vi "closed_loop.vi"() -> ()   [LabVIEW 2018]
uses:
  Controls/StatisticsData.ctl
  Classes/WavefrontCorrector/WavefrontCorrector.lvclass
  Classes/SlopesPostProcessorList/SlopesPostProcessorList.lvclass
  Classes/CorrectionDataManager/CorrectionDataManager.lvclass
  Classes/Camera/Camera.lvclass
  Classes/HasoEngine/HasoEngine.lvclass
  Classes/WavefrontCorrectorSet/WavefrontCorrectorSet.lvclass
  Classes/HasoData/HasoData.lvclass
  Classes/HasoSlopes/HasoSlopes.lvclass
  Classes/Image/Image.lvclass
  Classes/Phase/Phase.lvclass
  Classes/Pupil/Pupil.lvclass
  Classes/ComputePhaseSet/ComputePhaseSet.lvclass
  Classes/ClosedLoopSmoothing/ClosedLoopSmoothing.lvclass
  Controls/WavefrontReconstructionMode.ctl
  Controls/SlopesPostProcessorList - Filter.ctl
  Controls/InteractionMatrixToCommandMatrixParameters.ctl
panel:
  in  "init_state_from_config_file":bool
  out "Gain out":dbl min=0.0 max=1.0
  in  "Gain in":dbl min=0.0 max=1.0
  in  "Init":bool
  in  "Start Loop":bool
  in  "Exit":bool
  in  "Stop Loop":bool
  in  "error in (no error)":errorcluster
  out "Phase values":sgl[][](graph)
  out "Phase statistics":T1
  out "Camera image":u32[][](graph)
  in  "Interaction matrix file path":path
  out "error out":errorcluster
  out "ActuatorsNumber":i32
  in  "Wavefront configuration file path":path
  in  "Haso configuration file path":path
  # "This example is Hardware-dependant, \nplease use your own Haso and corrector configuration file and acquisition system, as well as your correction data backup file.\nIf you don't have a correction data backup file, please run the correction data example."
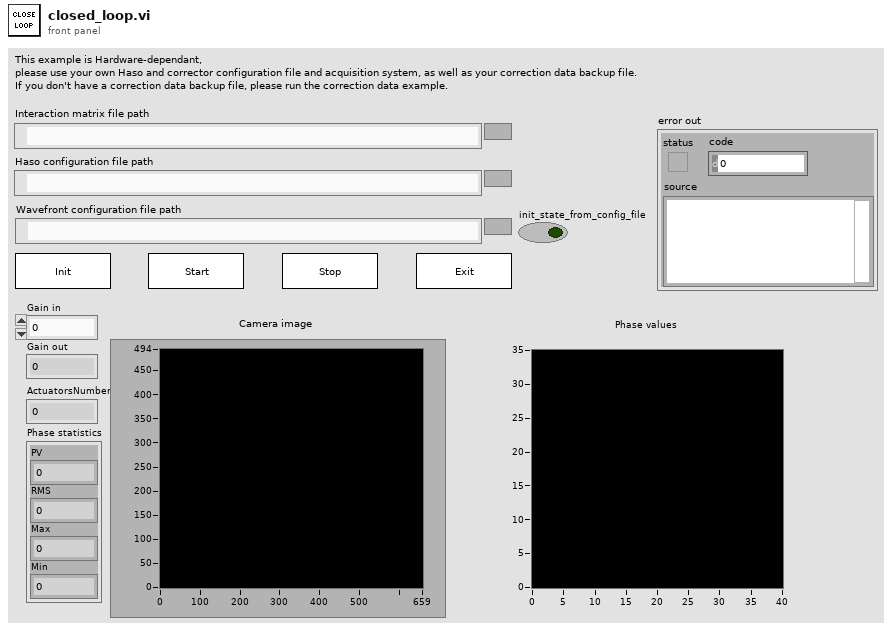
[diagram p1: front panel]
types:
  T1 = typedef "StatisticsData.ctl" = cluster{"PV":sgl, "RMS":dbl, "Max":sgl, "Min":sgl}
  T2 = typedef "WavefrontReconstructionMode.ctl" = enum16{"None", "Modal_Legendre", "Modal_Zernike", "Zonal", "Modal_Zonal_Zernike", "Modal_Zonal_Legendre"}
  T3 = typedef "SlopesPostProcessorList - Filter.ctl" = cluster{"tiltx":bool, "tilty":bool, "curv":bool, "astig0":bool, "astig45":bool, "others":bool}
  T4 = typedef "InteractionMatrixToCommandMatrixParameters.ctl" = cluster{"Number of kept modes":i32, "Tilt filtering":bool}
  T5 = typedef "CasaoManagerGeneralSpecifications.ctl" = cluster{"Wavefront corrector name":string, "Wavefront corrector serial number":string, "Nb actuators":i32, "HASO serial number":string, "Dimension_um":T6}
  T6 = typedef "General dimensions definition.ctl" = cluster{"Size":T7, "Step":T8}
  T7 = typedef "Point2D.ctl" = cluster{"X":u32, "Y":u32}
  T8 = typedef "Point2Df.ctl" = cluster{"X":sgl, "Y":sgl}
  T9 = typedef "Data alignment enum.ctl" = enum16{"8", "16", "32"}
  T10 = typedef "Wavefront Corrector states - ONE.ctl" = cluster{"Max":sgl, "Min":sgl, "Validity":enum16{"valid", "fixed", "invalid"}, "Fixed_Position":sgl}
  T11 = typedef "Wavefront Corrector Position.ctl" = sgl[]
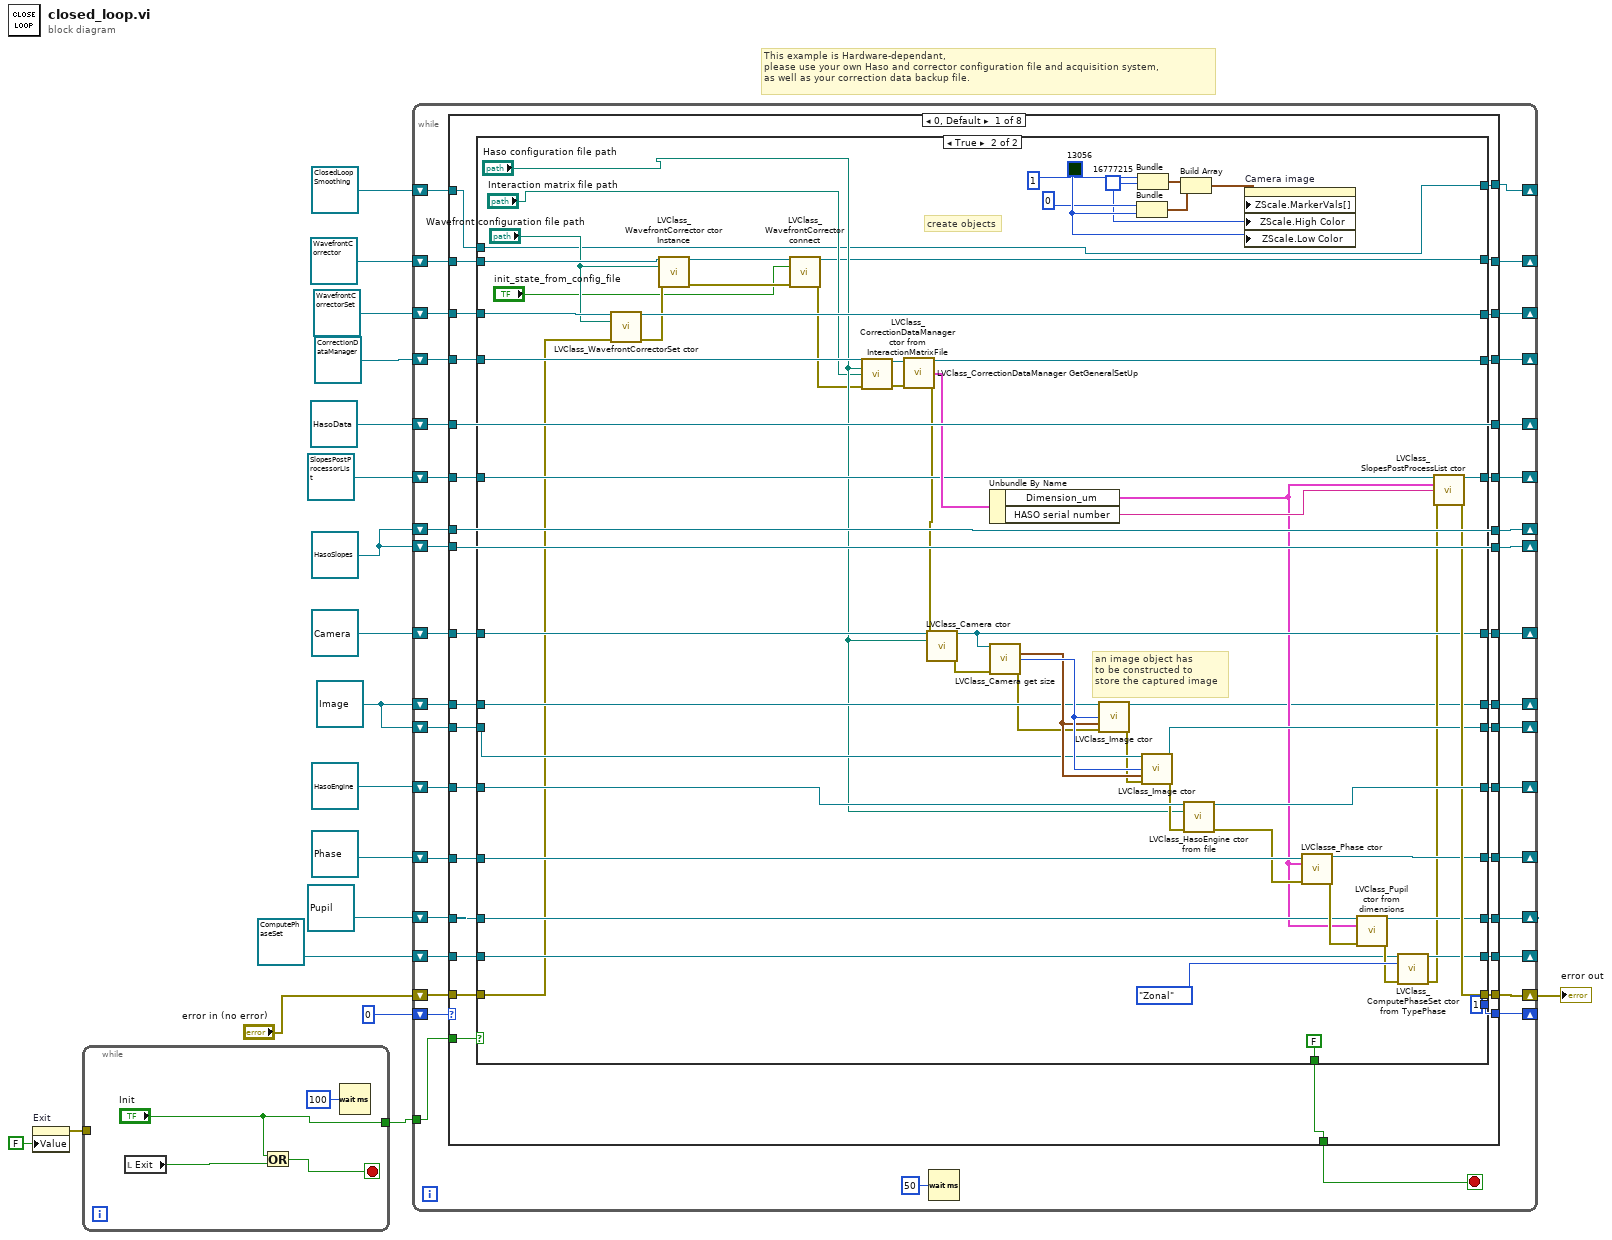
[diagram p0: block diagram]
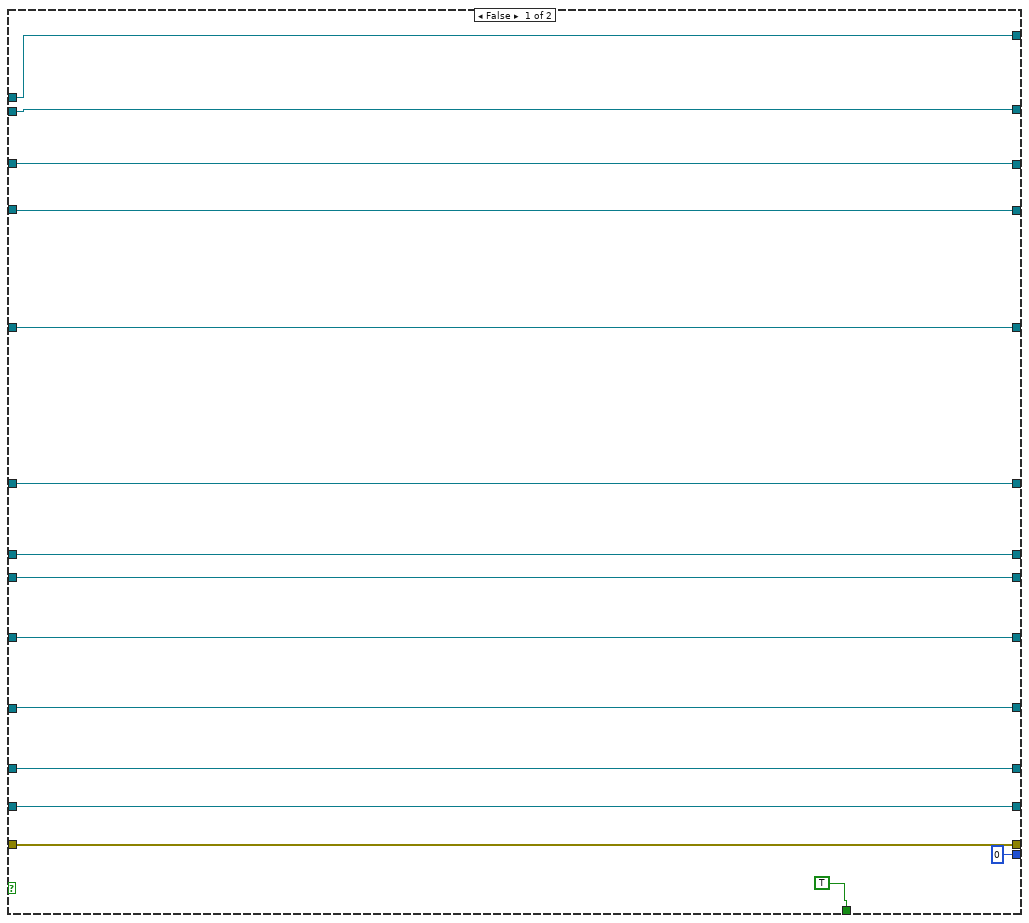
[diagram p2: hidden frame]
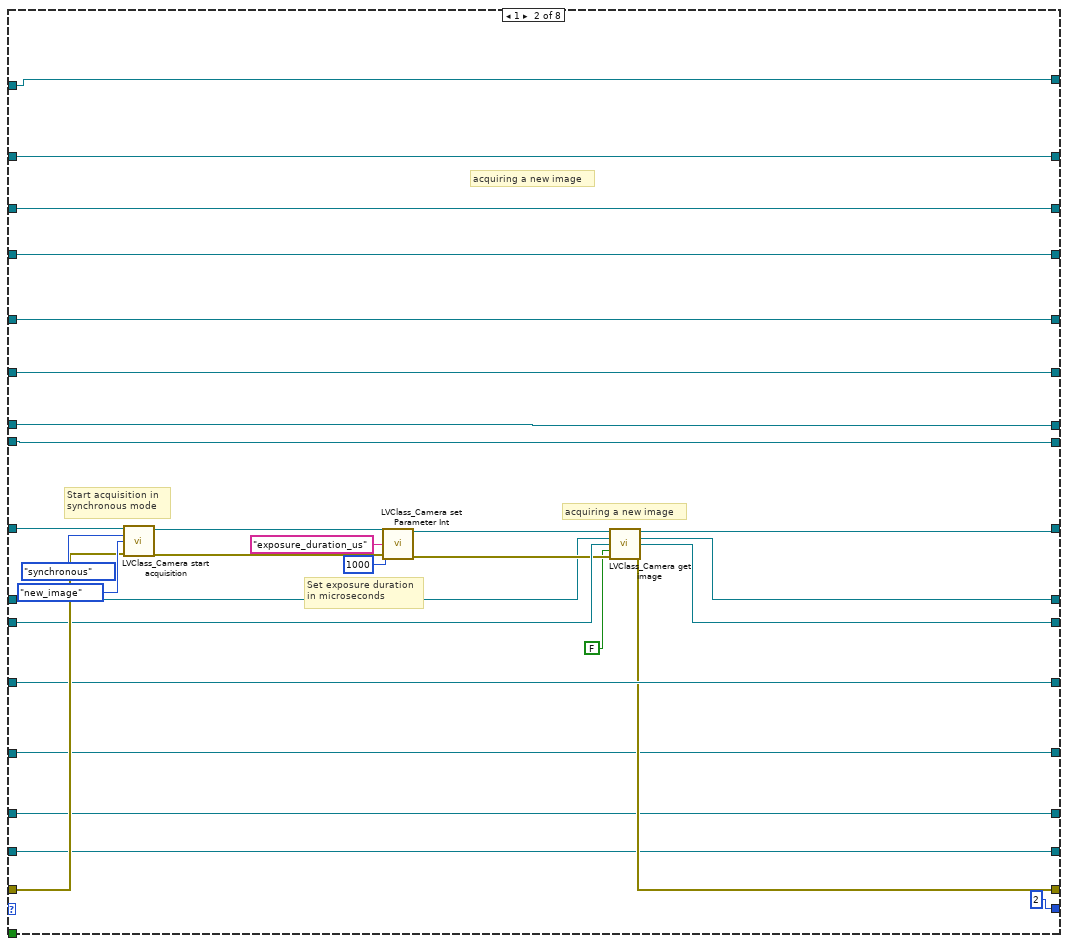
[diagram p3: hidden frame]
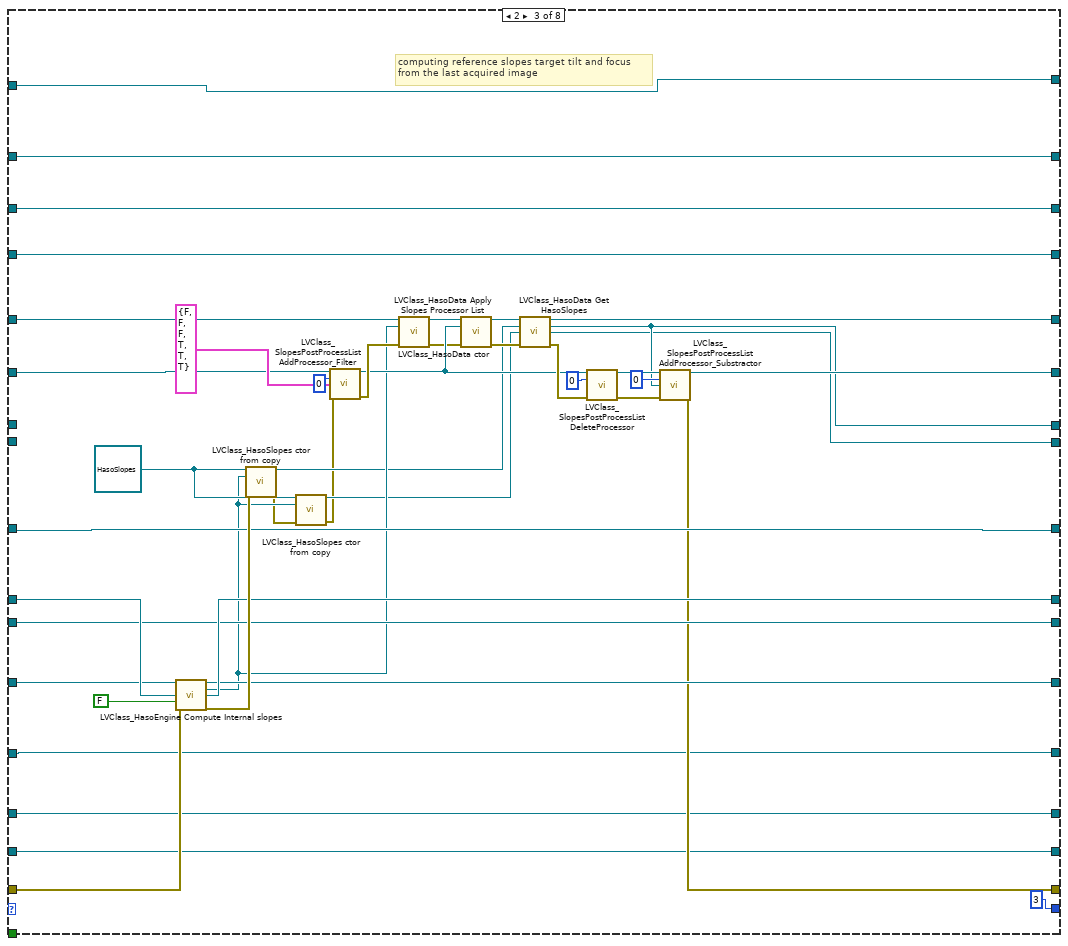
[diagram p4: hidden frame]
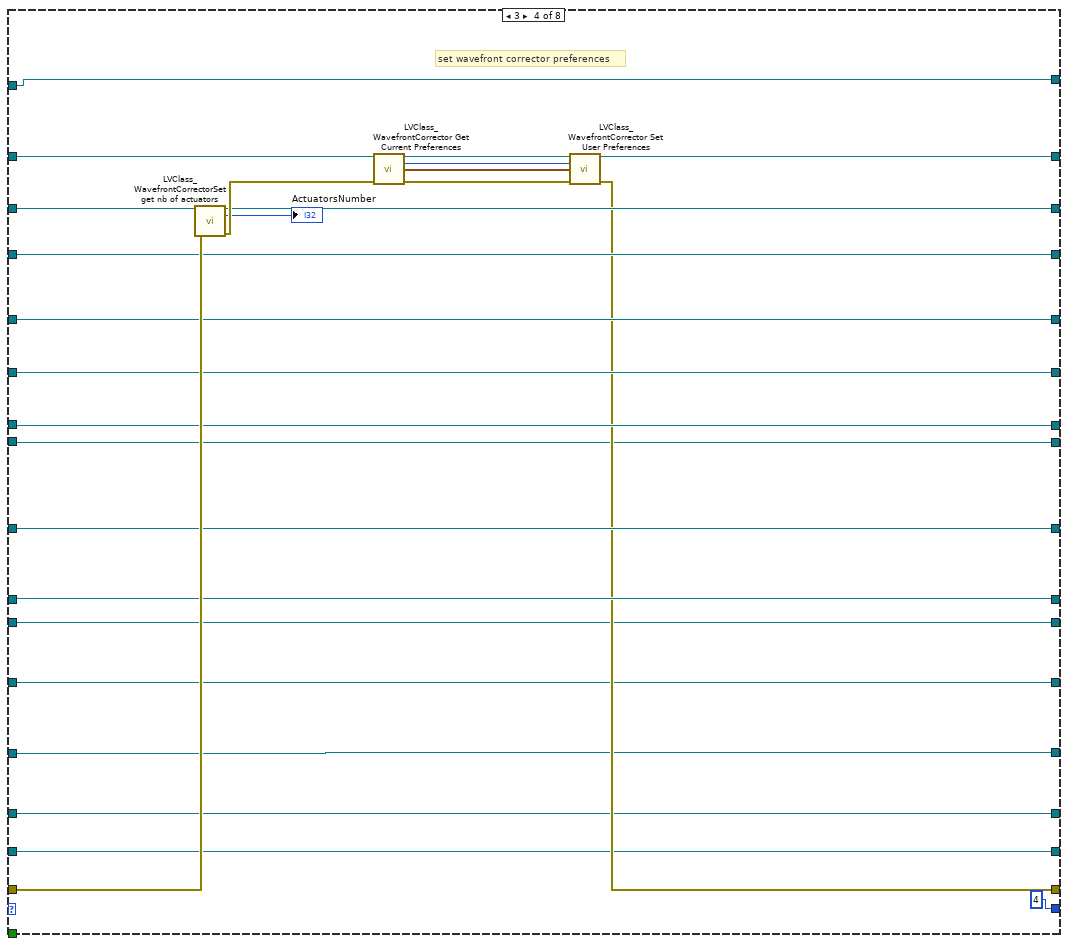
[diagram p5: hidden frame]
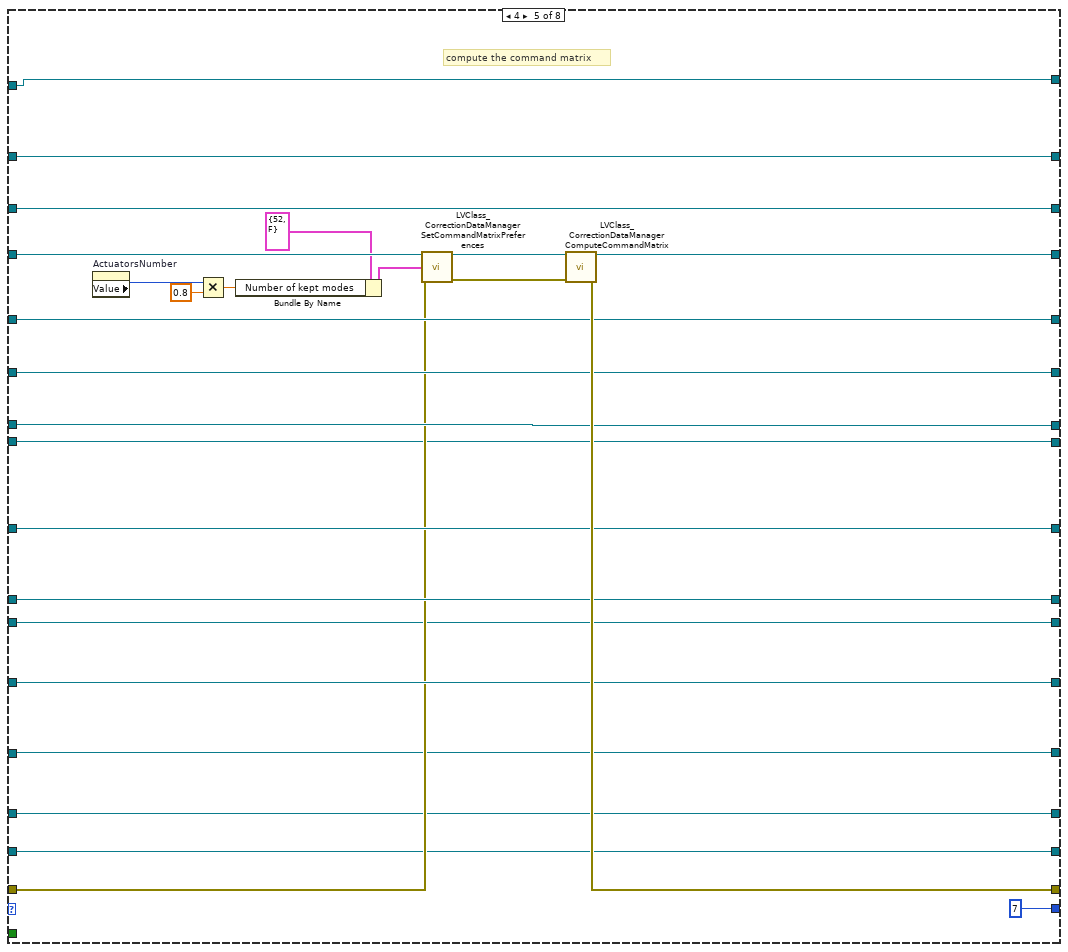
[diagram p6: hidden frame]
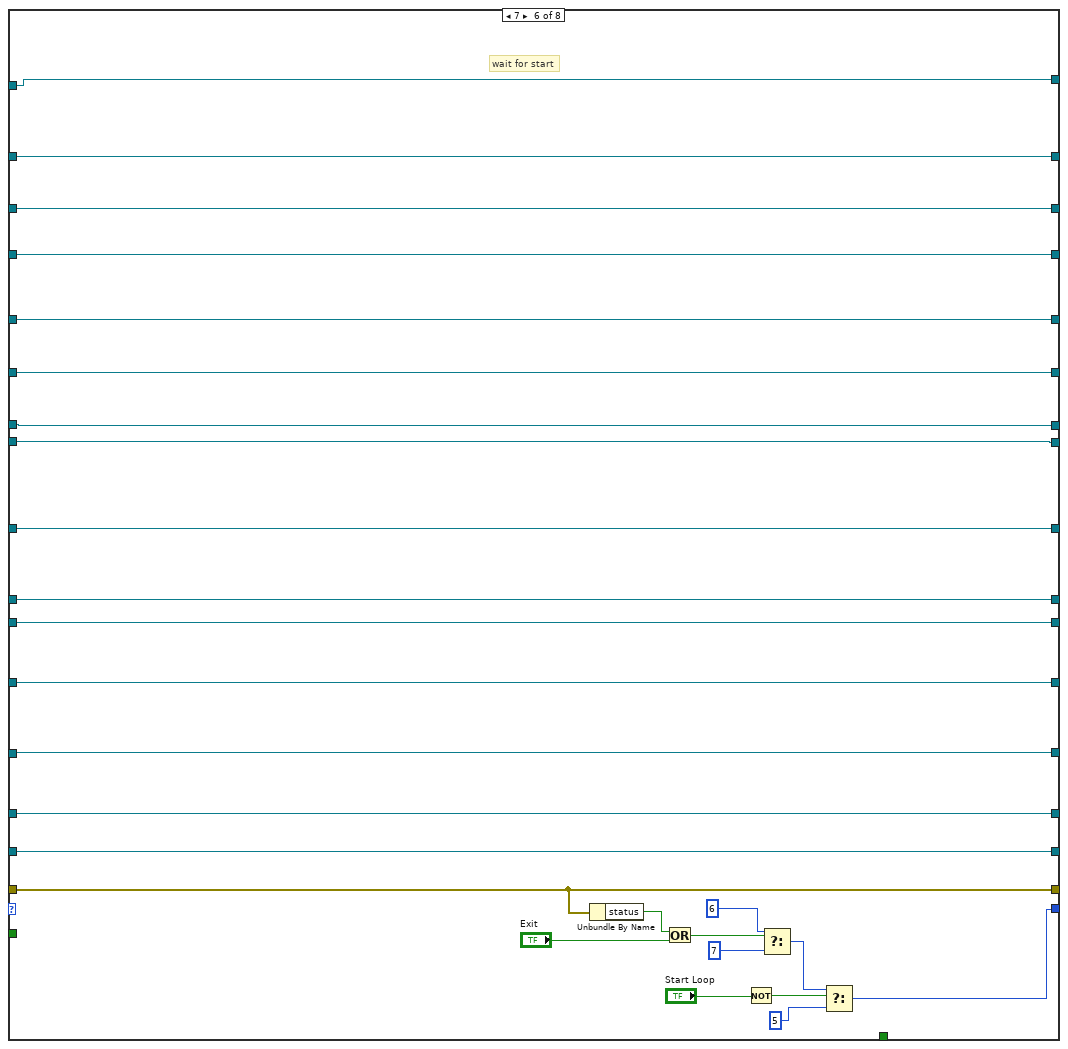
[diagram p7: hidden frame]
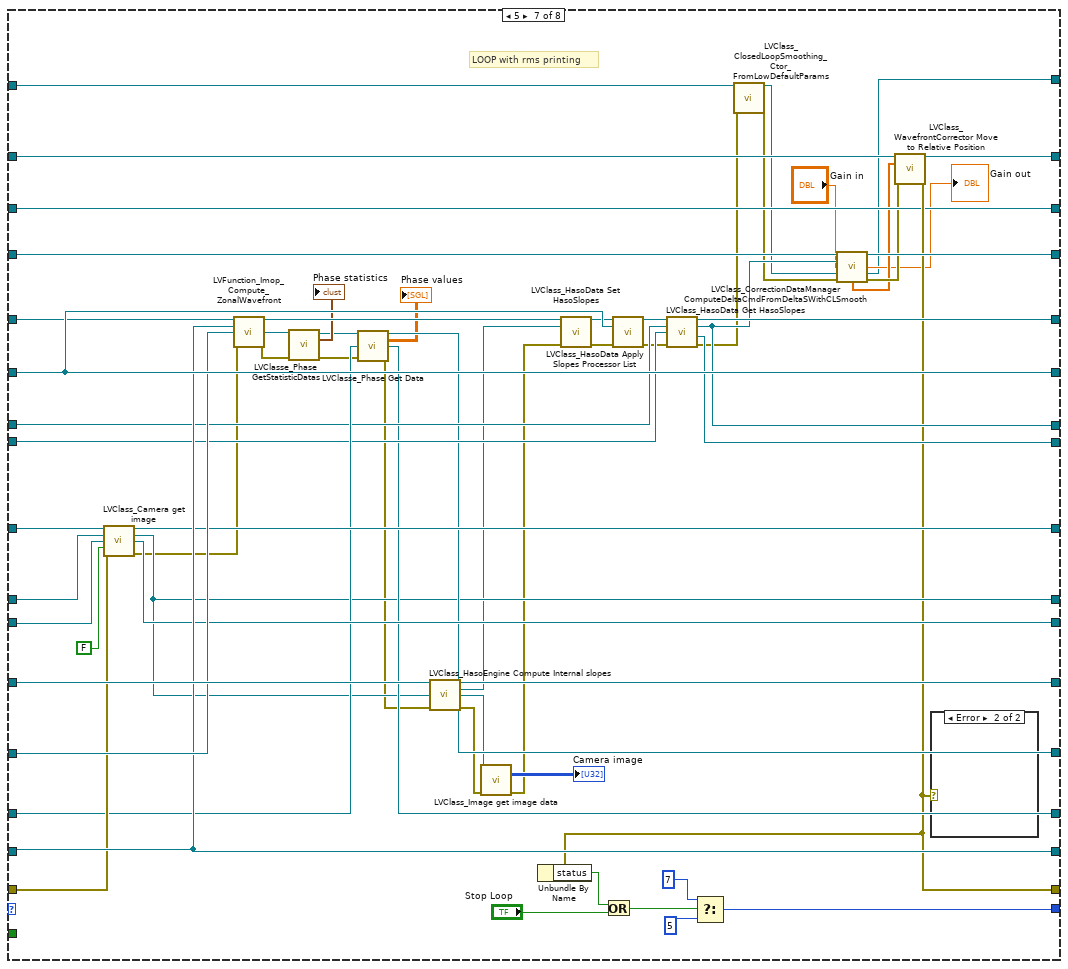
[diagram p8: hidden frame]
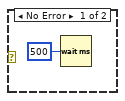
[diagram p9: hidden frame]
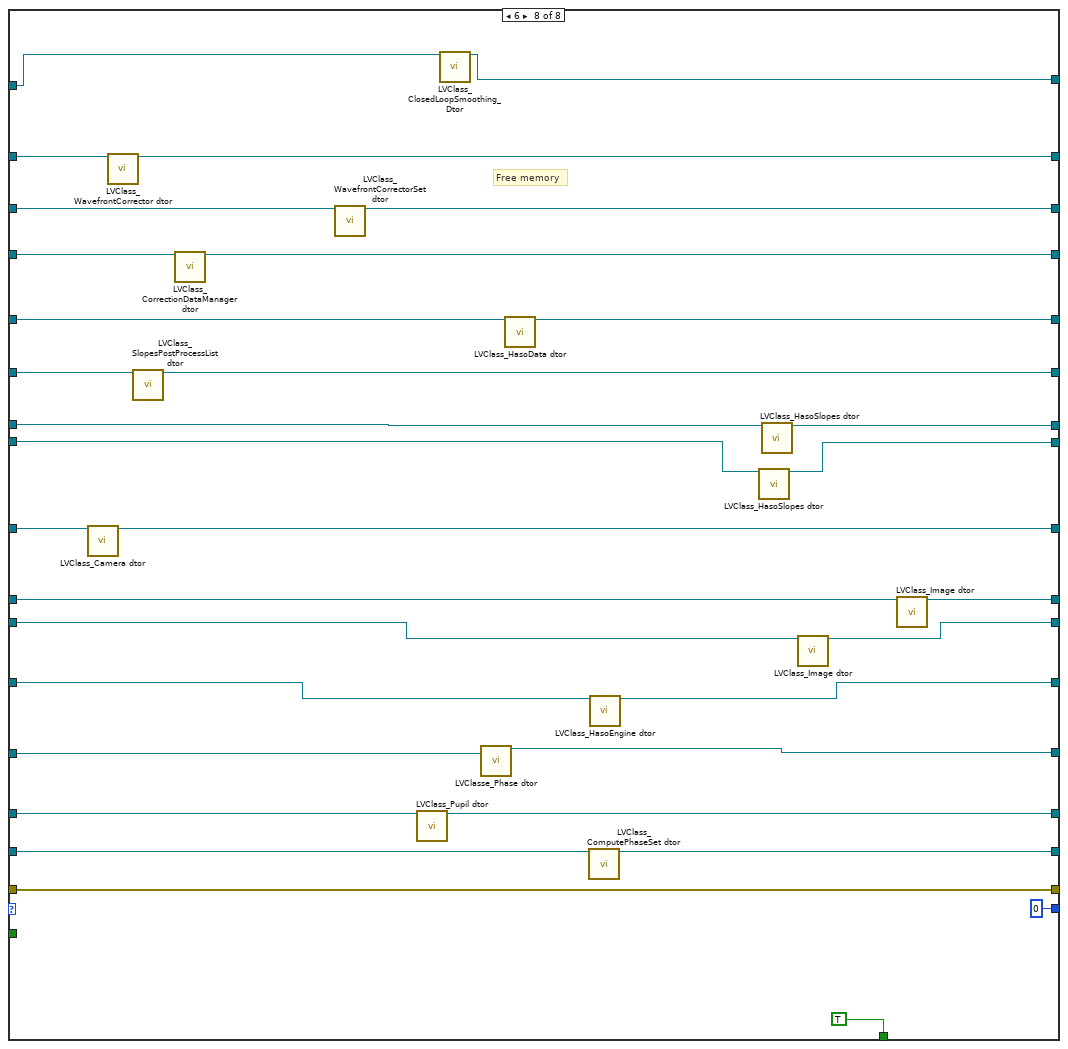
[diagram p10: hidden frame]
diagram:
  w10 = refnum<class "Image.lvclass"> refnum ("Image.lvclass")
  w6 = refnum<class "HasoSlopes.lvclass"> refnum ("HasoSlopes in")
  # "This example is Hardware-dependant, \nplease use your own Haso and corrector configuration file and acquisition system,\nas well as your correction data backup file."
  n1 = property on="Exit" class="Bool (strict)"("Value"=FALSE ("Exit")) -> (error out=w2:errorcluster)  [unwired: 2 in, 1 out]
  n2 = while {
    tunnel: ["Init"] -> w4
    tunnel: w2 -> [_]
    stop <- w21 stop-if-true
    n3 = local read "Exit"() -> (w22:bool)
    n4 = Or(x="Init", y=w22) -> (x .or. y?=w21:bool)
    n5 = Wait (ms)(milliseconds to wait=u32 100) -> ()  [unwired: 1 out]
  }
  n6 = while {
    shift-right: [w60] -> _
    shift-left: refnum<class "WavefrontCorrector.lvclass"> refnum ("WavefrontCorrector in") -> [w45]
    shift-right: [w57] -> _
    shift-left: refnum<class "CorrectionDataManager.lvclass"> refnum ("CorrectionDataManager in") -> [w44]
    shift-right: [w59] -> _
    shift-left: refnum<class "Camera.lvclass"> refnum ("Camera") -> [w54]
    shift-right: [w58] -> w11
    shift-left: "error in (no error)" -> [w53]
    shift-right: [w56] -> _
    shift-left: refnum<class "HasoEngine.lvclass"> refnum ("HasoEngine in") -> [w51]
    shift-right: [w55] -> _
    shift-left: refnum<class "SlopesPostProcessorList.lvclass"> refnum ("SlopesPostProcessorList in") -> [w49]
    shift-right: [w52] -> _
    shift-left: w10 -> [w50]
    shift-right: [w48] -> _
    shift-left: refnum<class "HasoData.lvclass"> refnum ("HasoData in") -> [w43]
    shift-right: [w47] -> _
    shift-left: refnum<class "WavefrontCorrectorSet.lvclass"> refnum ("WavefrontCorrectorSet in") -> [w46]
    shift-right: [w42] -> _
    shift-left: w6 -> [w41]
    shift-right: [w39] -> _
    shift-left: 0 -> [w38]
    shift-right: [w37] -> _
    shift-left: w10 -> [w36]
    shift-right: [w35] -> _
    shift-left: refnum<class "Phase.lvclass"> refnum ("Phase in") -> [w34]
    shift-right: [w33] -> _
    shift-left: refnum<class "Pupil.lvclass"> refnum ("Pupil in") -> [w32]
    shift-right: [w31] -> _
    shift-left: refnum<class "ComputePhaseSet.lvclass"> refnum ("ComputePhaseSet in") -> [w30]
    shift-right: [w29] -> _
    shift-left: w6 -> [w28]
    tunnel: w4 -> [w26]
    shift-right: [w24] -> _
    shift-left: refnum<class "ClosedLoopSmoothing.lvclass"> refnum ("ClosedLoopSmoothing.lvclass") -> [w25]
    stop <- w40 stop-if-true
    n7 = case shown="0, Default" w38 {
      tunnel: [w67 w186 w221 w259 w289 w317 w367 w403] -> w60
      tunnel: [w80 w188 w218 w251 w284 w310 w362 w397] -> w59
      tunnel: [w87 w173 w203 w250 w290 w300 w353 w392] -> w58
      tunnel: [w65 w183 w220 w254 w291 w315 w378 w400] -> w57
      tunnel: [w92 w181 w217 w249 w283 w307 w374 w396] -> w56
      tunnel: [w91 w185 w223 w256 w288 w313 w377 w402] -> w55
      tunnel: w54 -> [w84 w190 w218 w251 w284 w310 w373 w409]
      tunnel: w53 -> [w66 w189 w213 w264 w273 w300 w363 w392]
      tunnel: [w69 w179 w219 w252 w285 w309 w354 w398] -> w52
      tunnel: w51 -> [w83 w181 w212 w249 w283 w307 w375 w406]
      tunnel: w50 -> [w78 w175 w239 w252 w285 w309 w365 w404]
      tunnel: w49 -> [w86 w185 w225 w256 w288 w313 w377 w411]
      tunnel: [w81 w184 w210 w255 w287 w314 w376 w401] -> w48
      tunnel: [w90 w187 w222 w257 w282 w316 w352 w395] -> w47
      tunnel: w46 -> [w82 w187 w222 w265 w282 w316 w352 w405]
      tunnel: w45 -> [w68 w186 w221 w263 w289 w317 w368 w412]
      tunnel: w44 -> [w85 w183 w220 w254 w279 w315 w325 w408]
      tunnel: w43 -> [w81 w184 w215 w255 w287 w314 w370 w407]
      tunnel: [w89 w182 w202 w253 w286 w312 w357 w399] -> w42
      tunnel: w41 -> [w89 w182 _ w253 w286 w312 w360 w410]
      tunnel: [w63 _ _ _ _ _ _ TRUE] -> w40
      tunnel: [w88 2 3 4 7 w295 w372 0] -> w39
      tunnel: [w79 w174 w211 w247 w271 w308 w364 w390] -> w37
      tunnel: w36 -> [w77 w178 w211 w247 w271 w308 w366 w391]
      tunnel: [w76 w172 w199 w245 w269 w306 w355 w386] -> w35
      tunnel: w34 -> [w75 w172 w199 w245 w269 w306 w371 w388]
      tunnel: [w74 w171 w200 w244 w268 w305 w358 w385] -> w33
      tunnel: w32 -> [w73 w171 w200 w244 w268 w305 w361 w389]
      tunnel: [w72 w169 w198 w243 w267 w304 w369 w384] -> w31
      tunnel: w30 -> [w71 w169 w198 w243 w267 w304 w369 w387]
      tunnel: [w70 w170 w201 w246 w270 w311 w356 w382] -> w29
      tunnel: w28 -> [w70 w170 _ w246 w270 w311 w359 w383]
      tunnel: w26 -> [w64 _ _ _ _ _ _ _]
      tunnel: w25 -> [w62 w167 w197 w242 w266 w292 w322 w381]
      tunnel: [w61 w167 w197 w242 w266 w292 w318 w380] -> w24
      frame 0, Default {
        n8 = case shown="True" w64 {
          tunnel: [w97 w166] -> w92
          tunnel: [w101 w162] -> w91
          tunnel: [w103 w161] -> w90
          tunnel: [0 1] -> w88
          tunnel: [w107 w158] -> w87
          tunnel: w86 -> [w101 w157]
          tunnel: w85 -> [w102 w156]
          tunnel: w84 -> [w100 w155]
          tunnel: w83 -> [w97 w154]
          tunnel: w82 -> [w103 w153]
          tunnel: [w100 w152] -> w80
          tunnel: [w98 w149] -> w79
          tunnel: w78 -> [w99 w148]
          tunnel: w77 -> [w98 w147]
          tunnel: [w96 w142] -> w76
          tunnel: w75 -> [w96 w141]
          tunnel: [w95 w140] -> w74
          tunnel: w73 -> [w95 w138]
          tunnel: [w94 w134] -> w72
          tunnel: w71 -> [w94 w131]
          tunnel: [w99 w123] -> w69
          tunnel: w68 -> [w104 w122]
          tunnel: [w104 w111] -> w67
          tunnel: w66 -> [w107 w121]
          tunnel: [w102 w118] -> w65
          tunnel: [TRUE FALSE] -> w63
          tunnel: w62 -> [w93 w113]
          tunnel: [w93 w113] -> w61
          frame False {
          }
          frame True {
            w124 = u32 16777215
            w128 = u32 13056
            # "an image object has\nto be constructed to\nstore the captured image"
            # "create objects"
            n9 = call "LVClass_WavefrontCorrectorSet ctor.vi"("WavefrontCorrectorSet (const)"=w153, "PathToWavefrontCorrectorSetupFile"="Wavefront configuration file path", "error in (no error)"=w121) -> ("WavefrontCorrectorSet (new)"=w161:refnum<class "WavefrontCorrectorSet.lvclass">, "error out"=w120:errorcluster)  [unwired: 11 in]
            n10 = call "LVClass_WavefrontCorrector ctor Instance.vi"("WavefrontCorrector (const)"=w122, "PathToWavefrontCorrectorSetupFile"="Wavefront configuration file path", "error in (no error)"=w120) -> ("WavefrontCorrector (new)"=w112:refnum<class "WavefrontCorrector.lvclass">, "error out"=w110:errorcluster)  [unwired: 11 in]
            n11 = call "LVClass_WavefrontCorrector connect.vi"("WavefrontCorrector in"=w112, "set_init_state_from_config_file"="init_state_from_config_file", "error in (no error)"=w110) -> ("WavefrontCorrector out"=w111:refnum<class "WavefrontCorrector.lvclass">, "error out"=w109:errorcluster)  [unwired: 11 in]
            n12 = call "LVClass_CorrectionDataManager ctor from InteractionMatrixFile.vi"("CorrectionDataManager (const)"=w156, "Haso config file path"="Haso configuration file path", "Interaction matrix path"="Interaction matrix file path", "error in (no error)"=w109) -> ("CorrectionDataManager (new)"=w164:refnum<class "CorrectionDataManager.lvclass">, "error out"=w159:errorcluster)  [unwired: 10 in]
            n13 = call "LVClass_CorrectionDataManager GetGeneralSetUp.vi"("CorrectionDataManager in"=w164, "error in (no error)"=w159) -> ("CorrectionDataManager out"=w118:refnum<class "CorrectionDataManager.lvclass">, "general"=w165:T5, "error out"=w119:errorcluster)  [unwired: 11 in]
            n14 = call "LVClass_Camera ctor.vi"("Camera (const)"=w155, "Configuration file path"="Haso configuration file path", "error in (no error)"=w119) -> ("Camera (new)"=w152:refnum<class "Camera.lvclass">, "error out"=w144:errorcluster)  [unwired: 11 in]
            n15 = Unbundle By Name(w165) -> ("Dimension_um"=w136:T6, "HASO serial number"=w163:string)
            n16 = call "LVClass_Camera get size.vi"("Camera in"=w152, "error in (no error)"=w144) -> ("size"=w150:T7, "Number of bits"=w151:T9, "error out"=w146:errorcluster)  [unwired: 10 in, 1 out]
            n17 = call "LVClass_Image ctor.vi"("Image (const)"=w148, "Data alignment"=w151, "Size"=w150, "error in (no error)"=w146) -> ("Image (new)"=w123:refnum<class "Image.lvclass">, "error out"=w145:errorcluster)  [unwired: 10 in]
            n18 = Bundle(0, w128) -> (w129:cluster{i32, u32})  [unwired: 1 in]
            n19 = Bundle(1, w124) -> (w130:cluster{i32, u32})  [unwired: 1 in]
            n20 = call "LVClass_Image ctor.vi"("Image (const)"=w147, "Data alignment"=w151, "Size"=w150, "error in (no error)"=w145) -> ("Image (new)"=w149:refnum<class "Image.lvclass">, "error out"=w143:errorcluster)  [unwired: 10 in]
            n21 = Build Array(w130, w129) -> (w127:cluster{i32, u32}[])
            n22 = call "LVClass_HasoEngine ctor from file.vi"("HasoEngine (const)"=w154, "Configuration file path"="Haso configuration file path", "error in (no error)"=w143) -> ("HasoEngine (new)"=w166:refnum<class "HasoEngine.lvclass">, "error out"=w137:errorcluster)  [unwired: 11 in]
            n23 = property on="Camera image" class="IntGraph (strict)"("ZScale.MarkerVals[]"=w127, "ZScale.High Color"=w124, "ZScale.Low Color"=w128) -> ()  [unwired: 2 in, 2 out]
            n24 = call "LVClasse_Phase ctor.vi"("Phase (const)"=w141, "Dimensions_um"=w136, "error in (no error)"=w137) -> ("Phase (new)"=w142:refnum<class "Phase.lvclass">, "error out"=w139:errorcluster)  [unwired: 11 in]
            n25 = call "LVClass_Pupil ctor from dimensions.vi"("Pupil (const)"=w138, "Dimensions_um"=w136, "error in (no error)"=w139) -> ("Pupil (new)"=w140:refnum<class "Pupil.lvclass">, "error out"=w133:errorcluster)  [unwired: 11 in]
            n26 = call "LVClass_ComputePhaseSet ctor from TypePhase.vi"("ComputePhaseSet (const)"=w131, "TypePhase"=WavefrontReconstructionMode."Zonal", "error in (no error)"=w133) -> ("ComputePhaseSet (new)"=w134:refnum<class "ComputePhaseSet.lvclass">, "error out"=w132:errorcluster)  [unwired: 11 in]
            n27 = call "LVClass_SlopesPostProcessList ctor.vi"("SlopesPostProcessorList (const)"=w157, "Dimensions_um"=w136, "serial"=w163, "error in (no error)"=w132) -> ("SlopesPostProcessorList (new)"=w162:refnum<class "SlopesPostProcessorList.lvclass">, "error out"=w158:errorcluster)  [unwired: 10 in]
          }
        }
      }
      frame 1 {
        # "acquiring a new image"
        # "acquiring a new image"
        # "Set exposure duration\nin microseconds"
        # "Start acquisition in\nsynchronous mode"
        n28 = call "LVClass_Camera start acquisition.vi"("Camera in"=w190, "synchronisation_mode"=enum16{"synchronous", "asynchronous"}."synchronous", "acquisition_mode"=enum16{"last_image", "new_image"}."new_image", "error in (no error)"=w189) -> ("Camera out"=w195:refnum<class "Camera.lvclass">, "error out"=w196:errorcluster)  [unwired: 10 in]
        n29 = call "LVClass_Camera set Parameter Int.vi"("Camera in"=w195, "parameter_name"="exposure_duration_us", "value"=1000, "error in (no error)"=w196) -> ("Camera out"=w177:refnum<class "Camera.lvclass">, "error out"=w176:errorcluster)  [unwired: 10 in]
        n30 = call "LVClass_Camera get image.vi"("Camera in"=w177, "Image"=w175, "Image RAW"=w178, "remove_background"=FALSE, "error in (no error)"=w176) -> ("Camera out"=w188:refnum<class "Camera.lvclass">, "Image (dup)"=w179:refnum<class "Image.lvclass">, "Image (dup) RAW"=w174:refnum<class "Image.lvclass">, "error out"=w173:errorcluster)  [unwired: 7 in]
      }
      frame 2 {
        w209 = refnum<class "HasoSlopes.lvclass"> refnum ("HasoSlopes in")
        # "computing reference slopes target tilt and focus\nfrom the last acquired image"
        n31 = call "LVClass_HasoEngine Compute Internal slopes.vi"("HasoEngine in"=w212, "Image.lvclass"=w239, "learn_from_trimmer"=FALSE, "error in (no error)"=w213) -> ("HasoEngine out"=w217:refnum<class "HasoEngine.lvclass">, "HasoSlopes (dup)"=w208:refnum<class "HasoSlopes.lvclass">, "Image (dup)"=w219:refnum<class "Image.lvclass">, "error out"=w224:errorcluster)  [unwired: 7 in, 1 out]
        n32 = call "LVClass_HasoSlopes ctor from copy.vi"("HasoSlopes (const)"=w209, "HasoSlopes ToCopy"=w208, "error in (no error)"=w224) -> ("HasoSlopes (new)"=w207:refnum<class "HasoSlopes.lvclass">, "error out"=w205:errorcluster)  [unwired: 10 in, 1 out]
        n33 = call "LVClass_HasoSlopes ctor from copy.vi"("HasoSlopes (const)"=w209, "HasoSlopes ToCopy"=w208, "error in (no error)"=w205) -> ("HasoSlopes (new)"=w206:refnum<class "HasoSlopes.lvclass">, "error out"=w204:errorcluster)  [unwired: 10 in, 1 out]
        n34 = call "LVClass_SlopesPostProcessList AddProcessor_Filter.vi"("SlopesPostProcessorList in"=w225, "Position"=0, "Filter"=T3 {"tiltx"=FALSE, "tilty"=FALSE, "curv"=FALSE, "astig0"=TRUE, "astig45"=TRUE, "others"=TRUE}, "error in (no error)"=w204) -> ("SlopesPostProcessorList out"=w232:refnum<class "SlopesPostProcessorList.lvclass">, "error out"=w238:errorcluster)  [unwired: 10 in]
        n35 = call "LVClass_HasoData ctor.vi"("HasoData (const)"=w215, "HasoSlopes"=w208, "error in (no error)"=w238) -> ("HasoData (new)"=w228:refnum<class "HasoData.lvclass">, "error out"=w230:errorcluster)  [unwired: 10 in, 1 out]
        n36 = call "LVClass_HasoData Apply Slopes Processor List.vi"("HasoData in"=w228, "SlopesPostProcessorList"=w232, "error in (no error)"=w230) -> ("HasoData out"=w229:refnum<class "HasoData.lvclass">, "error out"=w231:errorcluster)  [unwired: 11 in]
        n37 = call "LVClass_HasoData Get HasoSlopes.vi"("HasoData in"=w229, "HasoSlopes"=w207, "HasoSlopes raw"=w206, "error in (no error)"=w231) -> ("HasoData out"=w210:refnum<class "HasoData.lvclass">, "HasoSlopes.dup"=w202:refnum<class "HasoSlopes.lvclass">, "HasoSlopes raw"=w201:refnum<class "HasoSlopes.lvclass">, "error out"=w236:errorcluster)  [unwired: 8 in]
        n38 = call "LVClass_SlopesPostProcessList DeleteProcessor.vi"("SlopesPostProcessorList in"=w232, "Position"=0, "error in (no error)"=w236) -> ("SlopesPostProcessorList out"=w234:refnum<class "SlopesPostProcessorList.lvclass">, "error out"=w237:errorcluster)  [unwired: 11 in]
        n39 = call "LVClass_SlopesPostProcessList AddProcessor_Substractor.vi"("SlopesPostProcessorList in"=w234, "Position"=0, "HasoSlopes.lvclass"=w202, "error in (no error)"=w237) -> ("SlopesPostProcessorList out"=w223:refnum<class "SlopesPostProcessorList.lvclass">, "error out"=w203:errorcluster)  [unwired: 10 in]
      }
      frame 3 {
        # "set wavefront corrector preferences"
        n40 = call "LVClass_WavefrontCorrectorSet get nb of actuators.vi"("WavefrontCorrectorSet in"=w265, "error in (no error)"=w264) -> ("WavefrontCorrectorSet out"=w257:refnum<class "WavefrontCorrectorSet.lvclass">, "ActuatorsNumber"=→"ActuatorsNumber":i32, "error out"=w262:errorcluster)  [unwired: 11 in]
        n41 = call "LVClass_WavefrontCorrector Get Current Preferences.vi"("WavefrontCorrector in"=w263, "error in (no error)"=w262) -> ("WavefrontCorrector out"=w261:refnum<class "WavefrontCorrector.lvclass">, "sleep_after_movement"=w241:i32, "Mirror preferences.Wavefront Corrector State"=w240:T10[], "error out"=w260:errorcluster)  [unwired: 10 in]
        n42 = call "LVClass_WavefrontCorrector Set User Preferences.vi"("WavefrontCorrector in"=w261, "Sleep after command apply_ms"=w241, "Wavefront Corrector State"=w240, "error in (no error)"=w260) -> ("WavefrontCorrector out"=w259:refnum<class "WavefrontCorrector.lvclass">, "error out"=w250:errorcluster)  [unwired: 10 in]
      }
      frame 4 {
        # "compute the command matrix"
        n43 = property on="ActuatorsNumber" class="DigNum (strict)"() -> ("Value"=w278:i32)  [unwired: 2 in, 2 out]
        n44 = Multiply(x=w278, y=0.8) -> (x*y=w275:dbl)
        n45 = Bundle By Name(cluster=T4 {"Number of kept modes"=52, "Tilt filtering"=FALSE} ("Prefs"), "Number of kept modes"=w275) -> (w274:T4)
        n46 = call "LVClass_CorrectionDataManager SetCommandMatrixPreferences.vi"("CorrectionDataManager in"=w279, "Prefs"=w274, "error in (no error)"=w273) -> ("CorrectionDataManager out"=w280:refnum<class "CorrectionDataManager.lvclass">, "error out"=w272:errorcluster)  [unwired: 11 in]
        n47 = call "LVClass_CorrectionDataManager ComputeCommandMatrix.vi"("CorrectionDataManager in"=w280, "error in (no error)"=w272) -> ("CorrectionDataManager out"=w291:refnum<class "CorrectionDataManager.lvclass">, "error out"=w290:errorcluster)  [unwired: 12 in]
      }
      frame 7 {
        # "wait for start"
        n48 = Unbundle By Name(w300) -> ("status"=w297:bool)
        n49 = Or(x=w297, y="Exit") -> (x .or. y?=w301:bool)
        n50 = Not(x="Start Loop") -> (.not. x?=w293:bool)
        n51 = Select(t=6, s=w301, f=7) -> (s? t:f=w296:i32)
        n52 = Select(t=w296, s=w293, f=5) -> (s? t:f=w295:i32)
      }
      frame 5 {
        # "LOOP with rms printing"
        n53 = call "LVClass_Camera get image.vi"("Camera in"=w373, "Image"=w365, "Image RAW"=w366, "remove_background"=FALSE, "error in (no error)"=w363) -> ("Camera out"=w362:refnum<class "Camera.lvclass">, "Image (dup)"=w354:refnum<class "Image.lvclass">, "Image (dup) RAW"=w364:refnum<class "Image.lvclass">, "error out"=w341:errorcluster)  [unwired: 7 in]
        n54 = call "LVFunction_Imop_Compute_ZonalWavefront.vi"("HasoData.lvclass"=w370, "ComputePhaseSet.lvclass"=w369, "Phase"=w371, "error constant"=w341) -> ("HasoData.lvclass (dup)"=w348:refnum<class "HasoData.lvclass">, "Phase"=w349:refnum<class "Phase.lvclass">, "error out"=w337:errorcluster)  [unwired: 8 in, 1 out]
        n55 = call "LVClasse_Phase GetStatisticDatas.vi"("Phase in"=w349, "error in (no error)"=w337) -> ("Phase out"=w335:refnum<class "Phase.lvclass">, "StatisticsData"=→"Phase statistics":T1, "error out"=w338:errorcluster)  [unwired: 11 in]
        n56 = call "LVClasse_Phase Get Data.vi"("Phase in"=w335, "Pupil"=w361, "error in (no error)"=w338) -> ("Phase out"=w355:refnum<class "Phase.lvclass">, "data"=→"Phase values":sgl[][], "Pupil (dup)"=w358:refnum<class "Pupil.lvclass">, "error out"=w336:errorcluster)  [unwired: 9 in]
        n57 = call "LVClass_HasoEngine Compute Internal slopes.vi"("HasoEngine in"=w375, "Image.lvclass"=w354, "error in (no error)"=w336) -> ("HasoEngine out"=w374:refnum<class "HasoEngine.lvclass">, "HasoSlopes (dup)"=w347:refnum<class "HasoSlopes.lvclass">, "Image (dup)"=w340:refnum<class "Image.lvclass">, "error out"=w339:errorcluster)  [unwired: 8 in, 1 out]
        n58 = call "LVClass_Image get image data.vi"("Image in"=w340, "error in (no error)"=w339) -> ("Image data out"=→"Camera image":u32[][], "error out"=w326:errorcluster)  [unwired: 11 in, 1 out]
        n59 = call "LVClass_HasoData Set HasoSlopes.vi"("HasoData"=w348, "HasoSlopes raw"=w347, "error in (no error)"=w326) -> ("HasoData out (dup)"=w346:refnum<class "HasoData.lvclass">, "error out"=w343:errorcluster)  [unwired: 10 in, 1 out]
        n60 = call "LVClass_HasoData Apply Slopes Processor List.vi"("HasoData in"=w346, "SlopesPostProcessorList"=w377, "error in (no error)"=w343) -> ("HasoData out"=w345:refnum<class "HasoData.lvclass">, "error out"=w344:errorcluster)  [unwired: 11 in]
        n61 = call "LVClass_HasoData Get HasoSlopes.vi"("HasoData in"=w345, "HasoSlopes"=w360, "HasoSlopes raw"=w359, "error in (no error)"=w344) -> ("HasoData out"=w376:refnum<class "HasoData.lvclass">, "HasoSlopes.dup"=w357:refnum<class "HasoSlopes.lvclass">, "HasoSlopes raw"=w356:refnum<class "HasoSlopes.lvclass">, "error out"=w321:errorcluster)  [unwired: 8 in]
        n62 = call "LVClass_ClosedLoopSmoothing_Ctor_FromLowDefaultParams.vi"("ClosedLoopSmoothing in"=w322, "error in (no error)"=w321) -> ("ClosedLoopSmoothing out"=w319:refnum<class "ClosedLoopSmoothing.lvclass">, "error out"=w320:errorcluster)  [unwired: 12 in]
        n63 = call "LVClass_CorrectionDataManager ComputeDeltaCmdFromDeltaSWithCLSmooth.vi"("CorrectionDataManager in"=w325, "Delta Slopes IN"=w357, "Gain in"="Gain in", "ClosedLoopSmoothing in"=w319, "error in (no error)"=w320) -> ("CorrectionDataManager out"=w378:refnum<class "CorrectionDataManager.lvclass">, "Gain out"=→"Gain out":dbl, "ClosedLoopSmoothing out"=w318:refnum<class "ClosedLoopSmoothing.lvclass">, "DeltaPosition"=w333:T11, "error out"=w334:errorcluster)  [unwired: 5 in, 1 out]
        n64 = call "LVClass_WavefrontCorrector Move to Relative Position.vi"("WavefrontCorrector in"=w368, "Wavefront Relative Position"=w333, "error in (no error)"=w334) -> ("WavefrontCorrector out"=w367:refnum<class "WavefrontCorrector.lvclass">, "error out"=w353:errorcluster)  [unwired: 11 in]
        n65 = Unbundle By Name(w353) -> ("status"=w330:bool)
        n66 = Or(x=w330, y="Stop Loop") -> (x .or. y?=w329:bool)
        n67 = Select(t=7, s=w329, f=5) -> (s? t:f=w372:i32)
        n68 = case shown="Error" w353 {
          frame No Error {
            n69 = Wait (ms)(milliseconds to wait=u32 500) -> ()  [unwired: 1 out]
          }
          frame Error {
          }
        }
      }
      frame 6 {
        # "Free memory"
        n70 = call "LVClass_Camera dtor.vi"("Camera in"=w409) -> ("Camera out"=w397:refnum<class "Camera.lvclass">)  [unwired: 13 in, 1 out]
        n71 = call "LVClass_WavefrontCorrector dtor.vi"("WavefrontCorrector in"=w412) -> ("WavefrontCorrector out"=w403:refnum<class "WavefrontCorrector.lvclass">)  [unwired: 13 in, 1 out]
        n72 = call "LVClass_SlopesPostProcessList dtor.vi"("SlopesPostProcessorList in"=w411) -> ("SlopesPostProcessorList out"=w402:refnum<class "SlopesPostProcessorList.lvclass">)  [unwired: 13 in, 1 out]
        n73 = call "LVClass_CorrectionDataManager dtor.vi"("CorrectionDataManager in"=w408) -> ("CorrectionDataManager out"=w400:refnum<class "CorrectionDataManager.lvclass">)  [unwired: 13 in, 1 out]
        n74 = call "LVClass_WavefrontCorrectorSet dtor.vi"("WavefrontCorrectorSet in"=w405) -> ("WavefrontCorrectorSet out"=w395:refnum<class "WavefrontCorrectorSet.lvclass">)  [unwired: 13 in, 1 out]
        n75 = call "LVClass_Pupil dtor.vi"("Pupil in"=w389) -> ("Pupil out"=w385:refnum<class "Pupil.lvclass">)  [unwired: 13 in, 1 out]
        n76 = call "LVClass_ClosedLoopSmoothing_Dtor.vi"("ClosedLoopSmoothing in"=w381) -> ("ClosedLoopSmoothing out"=w380:refnum<class "ClosedLoopSmoothing.lvclass">)  [unwired: 13 in, 1 out]
        n77 = call "LVClasse_Phase dtor.vi"("Phase in"=w388) -> ("Phase out"=w386:refnum<class "Phase.lvclass">)  [unwired: 13 in, 1 out]
        n78 = call "LVClass_HasoData dtor.vi"("HasoData in"=w407) -> ("HasoData out"=w401:refnum<class "HasoData.lvclass">)  [unwired: 13 in, 1 out]
        n79 = call "LVClass_ComputePhaseSet dtor.vi"("ComputePhaseSet in"=w387) -> ("ComputePhaseSet out"=w384:refnum<class "ComputePhaseSet.lvclass">)  [unwired: 13 in, 1 out]
        n80 = call "LVClass_HasoEngine dtor.vi"("HasoEngine in"=w406) -> ("HasoEngine out"=w396:refnum<class "HasoEngine.lvclass">)  [unwired: 13 in, 1 out]
        n81 = call "LVClass_HasoSlopes dtor.vi"("HasoSlopes in"=w383) -> ("HasoSlopes out"=w382:refnum<class "HasoSlopes.lvclass">)  [unwired: 13 in, 1 out]
        n82 = call "LVClass_HasoSlopes dtor.vi"("HasoSlopes in"=w410) -> ("HasoSlopes out"=w399:refnum<class "HasoSlopes.lvclass">)  [unwired: 13 in, 1 out]
        n83 = call "LVClass_Image dtor.vi"("Image in"=w391) -> ("Image out"=w390:refnum<class "Image.lvclass">)  [unwired: 13 in, 1 out]
        n84 = call "LVClass_Image dtor.vi"("Image in"=w404) -> ("Image out"=w398:refnum<class "Image.lvclass">)  [unwired: 13 in, 1 out]
      }
    }
    n85 = Wait (ms)(milliseconds to wait=u32 50) -> ()  [unwired: 1 out]
  }
  "error out" <- w11
